vi "Scan On Alarm.vi"(5 "UpperLimit":dbl, 6 "SweepCount":i32 format="%.0g", 7 "AlarmOutput":i32 format="%.0g", 8 "error in (no error)":errorcluster {"code" format="%.0x"}, 9 "AlarmChannel":string, 10 "ChannelList":string, 11 "instrument handle":refnum<k15>) -> (0 "error out":errorcluster {"code" format="%.0x"}, 3 "instrument handle out":refnum<k15>)   [LabVIEW 2020, in "Keysight DAQ970.lvlib"]
doc: "Configures the instrument to scan when an alarm occurs on the specified channel, initiates the scan putting instrument in wait for trigger (alarm) state, and monitors the specified channel."
uses:
  Keysight DAQ970.lvlib
  KtDAQ970.dll
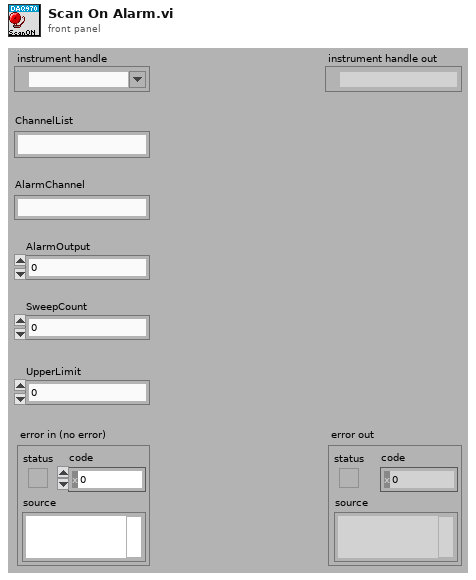
[diagram p1: front panel]
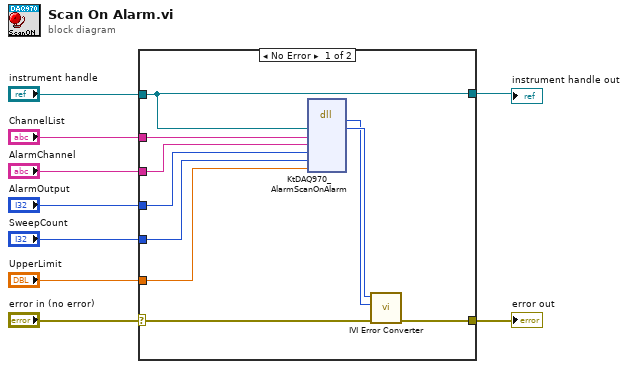
[diagram p0: block diagram]
diagram:
  n1 = case shown="No Error" "error in (no error)" {
    selector: "error in (no error)" -> [w17 w21]
    tunnel: [w16 w21] -> w9
    tunnel: "instrument handle" -> [w10 w20]
    tunnel: "ChannelList" -> [w15 _]
    tunnel: "AlarmChannel" -> [w14 _]
    tunnel: "AlarmOutput" -> [w13 _]
    tunnel: "SweepCount" -> [w12 _]
    tunnel: "UpperLimit" -> [w11 _]
    tunnel: [w10 w20] -> w1
    frame No Error {
      n2 = dll-call lib="KtDAQ970**.dll" fn="KtDAQ970_AlarmScanOnAlarm"("Vi"=w10, "ChannelList"=w15, "AlarmChannel"=w14, "AlarmOutput"=w13, "SweepCount"=w12, "UpperLimit"=w11) -> (w18:i32, "Vi"=w19:u32)  [unwired: 8 in, 2 out]
      n3 = call "IVI Error Converter.vi"("error in (no error)"=w17, "IVI error code (0)"=w18, "instrument handle"=w19) -> ("error out"=w16:errorcluster)  [unwired: 7 in, 1 out]
    }
    frame Error {
    }
  }
  "error out" <- w9
  "instrument handle out" <- w1
